vi "VG_WaveChart.vi"() -> ()   [LabVIEW 2020]
panel:
  in  "WaveChart":dbl=20.0
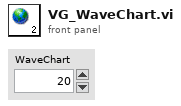
[diagram p1: front panel]
diagram:
